vi "AMC Dispatch Ping.vi"(8 "error in (no error)":errorcluster, 9 "Timeout (100 ms)":i32=100, 11 "receiver host":string) -> (0 "error out":errorcluster, 2 "String Response":string, 3 "Message":T1)   [LabVIEW 2017]
uses:
  Tools/Keyed Array/Tools_KeyedArray KeyedArray.ctl
  subVIs/TypeDefs/amc_Message.ctl
  subVIs/amc_Globals.vi
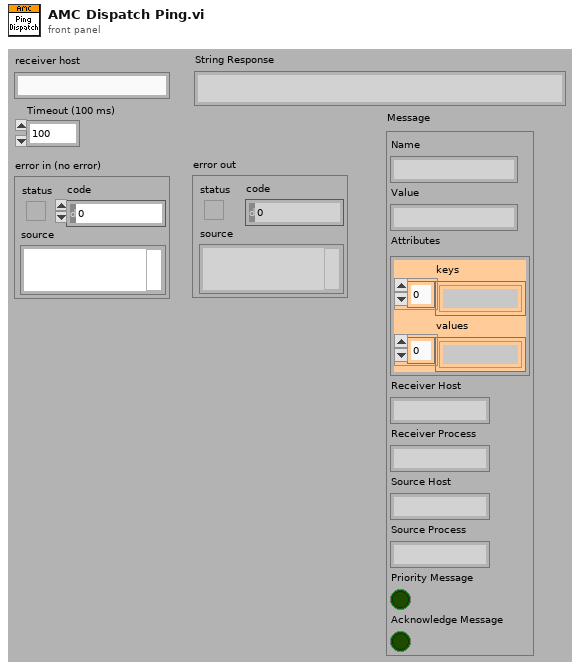
[diagram p1: front panel]
types:
  T1 = typedef "amc_Message.ctl" = cluster{"Name":string, "Value":string, "Attributes":T2, "Receiver Host":string, "Receiver Process":string, "Source Host":string, "Source Process":string, "Priority Message":bool, "Acknowledge Message":bool}
  T2 = typedef "Tools_KeyedArray KeyedArray.ctl" = cluster{"keys":string[], "values":string[]}
  T3 = typedef "amc_Message Queue.ctl" = refnum<queue>
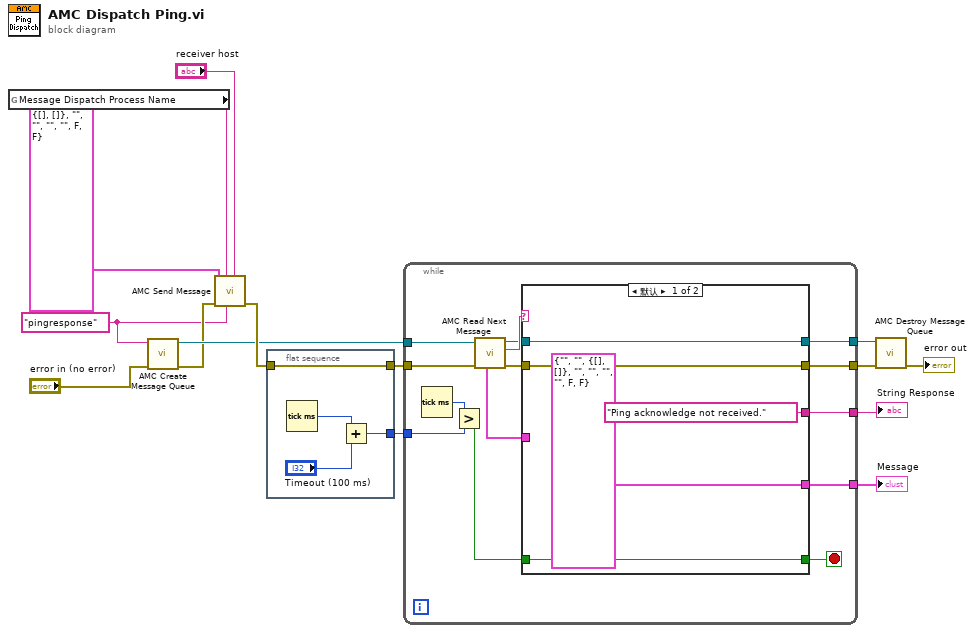
[diagram p0: block diagram]
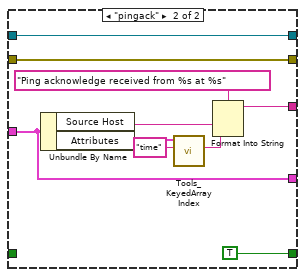
[diagram p2: hidden frame]
diagram:
  w3 = "pingresponse" ("message queue name")
  n1 = global read "amc_Globals.vi" "Message Dispatch Process Name"() -> (w1:string)
  n2 = call "AMC Create Message Queue.vi"("error in (no error)"="error in (no error)", "Message Queue Name"=w3) -> ("error out"=w4:errorcluster, "Message Queue out"=w5:T3)  [unwired: 2 in, 6 out]
  n3 = call "AMC Send Message.vi"("Receiver Host"="receiver host", "Source Process"=w3, "Receiver Process"=w1, "error in (no error)"=w4, "Message"=T1 {"Name"="ping", "Value"="", "Attributes"={"keys"=[], "values"=[]}, "Receiver Host"="", "Receiver Process"="", "Source Host"="", "Source Process"="", "Priority Message"=FALSE, "Acknowledge Message"=FALSE}) -> ("error out"=w10:errorcluster)  [unwired: 3 in, 3 out]
  n4 = flat-sequence {
    tunnel: [w19] -> w9
    tunnel: w10 -> [w19]
    tunnel: [w16] -> w8
    frame #0 {
      n5 = Tick Count (ms)() -> (millisecond timer value=w18:u32)
      n6 = Add(x=w18, y="Timeout (100 ms)") -> (x+y=w16:u32)
    }
  }
  n7 = while {
    tunnel: w9 -> [w33]
    tunnel: [w30] -> w13
    tunnel: [w29] -> w12
    tunnel: [w26] -> w6
    tunnel: [w25] -> w7
    tunnel: w5 -> [w24]
    tunnel: w8 -> [w22]
    stop <- w21 stop-if-true
    n8 = Tick Count (ms)() -> (millisecond timer value=w23:u32)
    n9 = Greater?(x=w23, y=w22) -> (0:w20:bool)
    n10 = call "AMC Read Next Message.vi"("error in (no error)"=w33, "Message Queue in"=w24) -> ("error out"=w28:errorcluster, "Message Name"=w32:string, "Message Queue out"=w27:T3, "Message"=w31:T1)  [unwired: 2 in, 4 out]
    n11 = case shown="默认" w32 {
      tunnel: w31 -> [_ w42]
      tunnel: ["Ping acknowledge not received." w43] -> w30
      tunnel: [T1 {"Name"="", "Value"="", "Attributes"={"keys"=[], "values"=[]}, "Receiver Host"="", "Receiver Process"="", "Source Host"="", "Source Process"="", "Priority Message"=FALSE, "Acknowledge Message"=FALSE} ("Message") w42] -> w29
      tunnel: [w35 w41] -> w26
      tunnel: w28 -> [w35 w41]
      tunnel: [w36 w40] -> w25
      tunnel: w27 -> [w36 w40]
      tunnel: [w34 TRUE] -> w21
      tunnel: w20 -> [w34 _]
      frame Default {
      }
      frame "pingack" {
        n12 = Unbundle By Name(w42) -> ("Source Host"=w48:string, "Attributes"=w45:T2)
        n13 = call "Tools_KeyedArray Index.vi"("key"="time", "array in"=w45) -> ("value"=w47:string)  [unwired: 2 in, 3 out]
        n14 = Format Into String(format string="Ping acknowledge received from %s at %s", w48, w47) -> (resulting string=w43:string)  [unwired: 2 in, 1 out]
      }
    }
  }
  "String Response" <- w13
  "Message" <- w12
  n15 = call "AMC Destroy Message Queue.vi"("error in (no error)"=w6, "Message Queue in"=w7) -> ("error out"=→"error out":errorcluster)  [unwired: 9 out]
